vi "_Buffer_To_AllElements.vi"(10 "count (-1: all)":i32=-1, 11 "Buffer":refnum<class "ObjectBuffer.lvclass">) -> (3 "Elements":refnum<class>[](array[class]))   [LabVIEW 2013]
uses:
  ObjectBuffer.lvclass
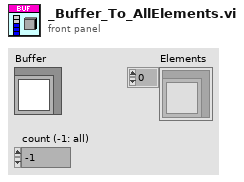
[diagram p1: front panel]
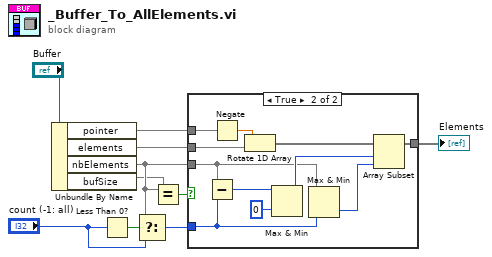
[diagram p0: block diagram]
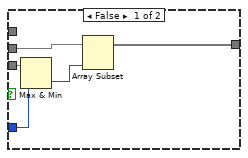
[diagram p2: hidden frame]
diagram:
  n1 = Unbundle By Name("Buffer") -> ("pointer"=w4, "elements"=w1, "nbElements"=w9, "bufSize"=w6)
  n2 = Less Than 0?(x="count (-1: all)") -> (x < 0?=w7:bool)
  n3 = Select(t=w9, s=w7, f="count (-1: all)") -> (s? t:f=w8:i32)
  n4 = Equal?(x=w9, y=w6) -> (x = y?=w5:bool)
  n5 = case shown="True" w5 {
    tunnel: w1 -> [w11 w26]
    tunnel: [w15 w24] -> w3
    tunnel: w8 -> [w12 w19]
    tunnel: w4 -> [_ w17]
    tunnel: w9 -> [w13 w16]
    frame False {
      n6 = Max & Min(x=w13, y=w12) -> (min(x,y)=w14:i32)  [unwired: 1 out]
      n7 = Array Subset(array=w11, length=w14) -> (w15:void[])  [unwired: 1 in]
    }
    frame True {
      n8 = Subtract(x=w16, y=w19) -> (x-y=w22:i32)
      n9 = Negate(x=w17) -> (-x=w23:dbl)
      n10 = Rotate 1D Array(1:w26, 2:w23) -> (0:w25:void[])
      n11 = Max & Min(x=w22, y=0) -> (max(x,y)=w20:i32)  [unwired: 1 out]
      n12 = Max & Min(x=w16, y=w19) -> (min(x,y)=w18:i32)  [unwired: 1 out]
      n13 = Array Subset(array=w25, index=w20, length=w18) -> (w24:void[])
    }
  }
  "Elements" <- w3
